vi "CAlex_InitConfig3DoF_test.vi"(8 "error in (no error)":errorcluster, 11 "C-Alex in":refnum<class "CableSerialChain.lvclass">) -> (0 "error out":errorcluster, 3 "C-Alex out":refnum<class "CableSerialChain.lvclass">)   [LabVIEW 2014]
uses:
  Body/Bodies.lvclass
  Body/PointOnBody.ctl
  Cable.ctl
  CableSerialChain.lvclass
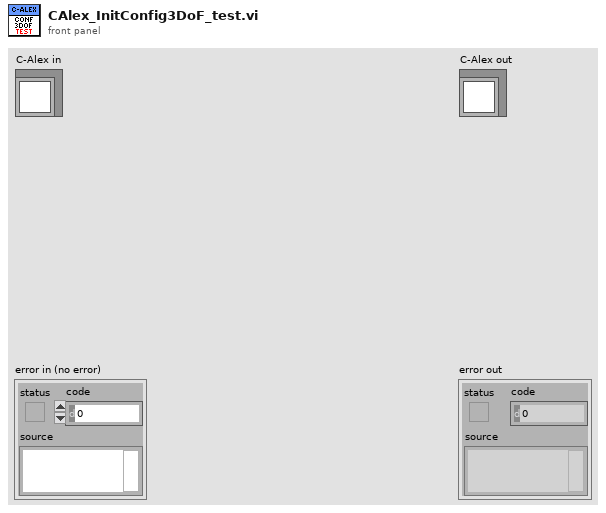
[diagram p1: front panel]
types:
  T1 = typedef "CableSerialChain.lvclass/Cable.ctl" = cluster{"RoutingPtsInLegCoSys":T2[], "Cable ID":i32}
  T2 = typedef "Bodies.lvclass/PointOnBody.ctl" = cluster{"Coord4":dbl[], "ID":i32}
  T3 = cluster{cluster{enum16{"Theta", "Alpha", "a", "d"}, dbl}[], "CoM_Pos":T2, "Mass(kg)":dbl}[]
  T4 = cluster{enum16{"Theta", "Alpha", "a", "d"}, dbl}[][]
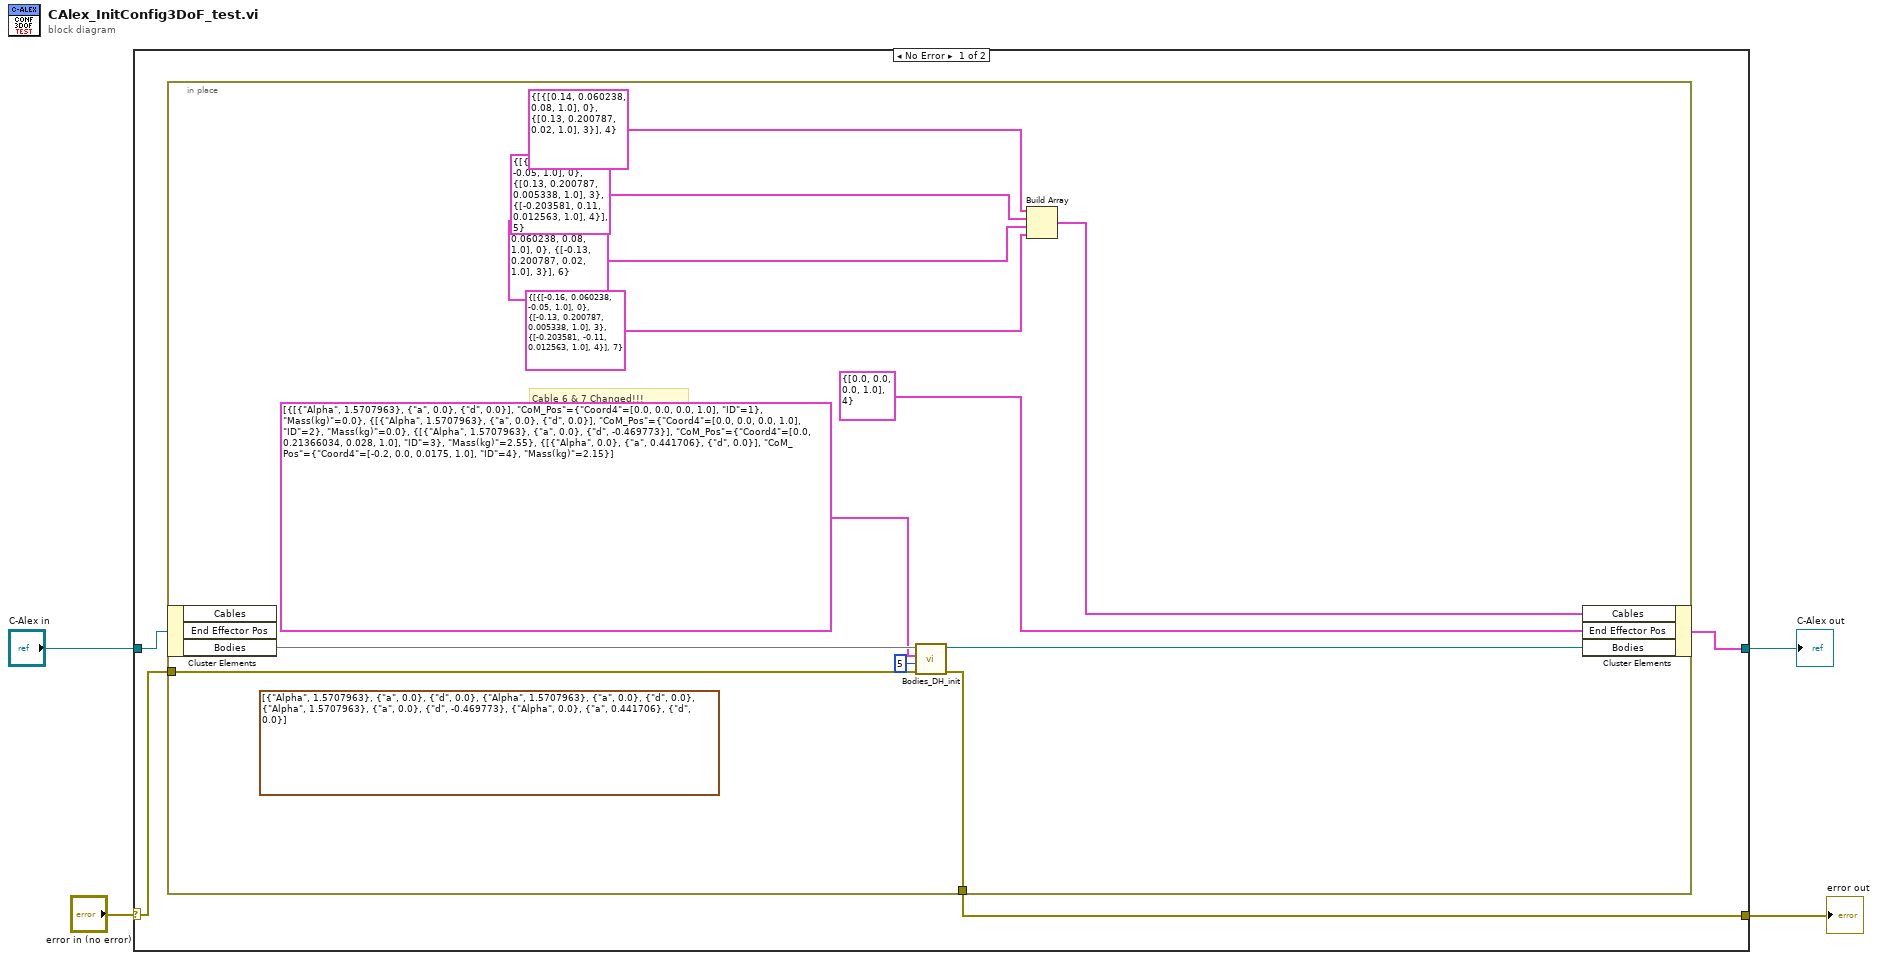
[diagram p0: block diagram]
diagram:
  n1 = case shown="No Error" "error in (no error)" {
    selector: "error in (no error)" -> [w7 w21]
    tunnel: [w5 w21] -> w3
    tunnel: [w6 w22] -> w1
    tunnel: "C-Alex in" -> [w8 w22]
    frame No Error {
      n2 = in-place {
        in-place-border: w7 -> [w19]
        in-place-border: [w16] -> w5
        (unwired) T4 [[{enum."Alpha", 1.5707963}, {enum."a", 0.0}, {enum."d", 0.0}], [{enum."Alpha", 1.5707963}, {enum."a", 0.0}, {enum."d", 0.0}], [{enum."Alpha", 1.5707963}, {enum."a", 0.0}, {enum."d", -0.469773}], [{enum."Alpha", 0.0}, {enum."a", 0.441706}, {enum."d", 0.0}]] ("KnownVar")
        # "Cable 6 & 7 Changed!!!"
        n3 = in-place-cluster #1(w8) -> ("Bodies"=w20)  [unwired: 2 out]
        n4 = call "Bodies_DH_init.vi"("error in (no error)"=w19, "Number of Bodies (Including Base)"=5, "KnownDHVars"=T3 [{[{enum."Alpha", 1.5707963}, {enum."a", 0.0}, {enum."d", 0.0}], "CoM_Pos"={"Coord4"=[0.0, 0.0, 0.0, 1.0], "ID"=1}, "Mass(kg)"=0.0}, {[{enum."Alpha", 1.5707963}, {enum."a", 0.0}, {enum."d", 0.0}], "CoM_Pos"={"Coord4"=[0.0, 0.0, 0.0, 1.0], "ID"=2}, "Mass(kg)"=0.0}, {[{enum."Alpha", 1.5707963}, {enum."a", 0.0}, {enum."d", -0.469773}], "CoM_Pos"={"Coord4"=[0.0, 0.21366034, 0.028, 1.0], "ID"=3}, "Mass(kg)"=2.55}, {[{enum."Alpha", 0.0}, {enum."a", 0.441706}, {enum."d", 0.0}], "CoM_Pos"={"Coord4"=[-0.2, 0.0, 0.0175, 1.0], "ID"=4}, "Mass(kg)"=2.15}], "Body.lvclass In"=w20) -> ("error out"=w16:errorcluster, "Body.lvclass Out"=w18:refnum<class "Bodies.lvclass">)  [unwired: 6 in]
        n5 = Build Array(T1 {"RoutingPtsInLegCoSys"=[{"Coord4"=[0.14, 0.060238, 0.08, 1.0], "ID"=0}, {"Coord4"=[0.13, 0.200787, 0.02, 1.0], "ID"=3}], "Cable ID"=4} ("Cable"), T1 {"RoutingPtsInLegCoSys"=[{"Coord4"=[0.16, 0.060238, -0.05, 1.0], "ID"=0}, {"Coord4"=[0.13, 0.200787, 0.005338, 1.0], "ID"=3}, {"Coord4"=[-0.203581, 0.11, 0.012563, 1.0], "ID"=4}], "Cable ID"=5} ("Cable"), T1 {"RoutingPtsInLegCoSys"=[{"Coord4"=[-0.14, 0.060238, 0.08, 1.0], "ID"=0}, {"Coord4"=[-0.13, 0.200787, 0.02, 1.0], "ID"=3}], "Cable ID"=6} ("Cable"), T1 {"RoutingPtsInLegCoSys"=[{"Coord4"=[-0.16, 0.060238, -0.05, 1.0], "ID"=0}, {"Coord4"=[-0.13, 0.200787, 0.005338, 1.0], "ID"=3}, {"Coord4"=[-0.203581, -0.11, 0.012563, 1.0], "ID"=4}], "Cable ID"=7} ("Cable")) -> (w11:T1[])
        n6 = in-place-cluster #1("Cables"=w11, "End Effector Pos"=T2 {"Coord4"=[0.0, 0.0, 0.0, 1.0], "ID"=4} ("Point"), "Bodies"=w18) -> (w6:cluster{})
      }
    }
    frame Error {
    }
  }
  "error out" <- w3
  "C-Alex out" <- w1
